vi "Is cancelled.vi"(8 "error in (no error)":errorcluster, 11 "Progress Dialog in":refnum<class "Progress Dialog.lvclass">) -> (0 "error out":errorcluster, 2 "Cancelled?":bool, 3 "Progress Dialog out":refnum<class "Progress Dialog.lvclass">)   [LabVIEW 2011, in "COSYLib.lvlib" / "Progress Dialog.lvclass"]
uses:
  Progress Dialog.lvclass
  Progress Dialog.lvclass/Progress Dialog.ctl
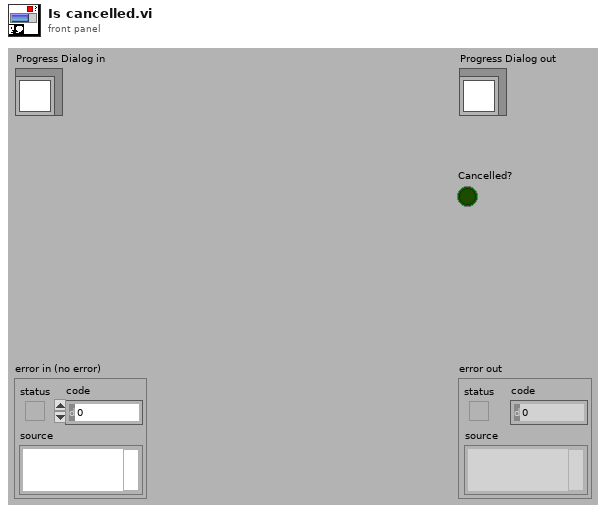
[diagram p1: front panel]
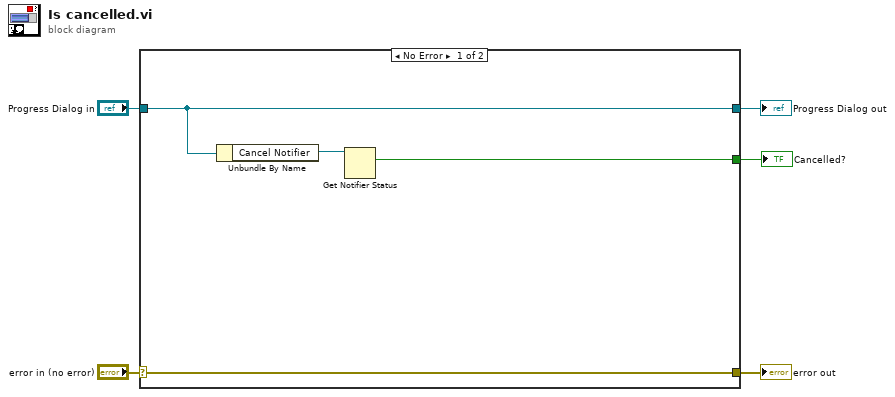
[diagram p0: block diagram]
diagram:
  n1 = case shown="No Error" "error in (no error)" {
    selector: "error in (no error)" -> [w9 w11]
    tunnel: [w9 w11] -> w4
    tunnel: [w8 w10] -> w2
    tunnel: "Progress Dialog in" -> [w8 w10]
    tunnel: [w6 _] -> w1
    frame No Error {
      n2 = Unbundle By Name(w8) -> ("Cancel Notifier"=w7:refnum<notifier>)
      n3 = Get Notifier Status(notifier=w7) -> (current notification=w6:bool)  [unwired: 1 in, 4 out]
    }
    frame Error {
    }
  }
  "error out" <- w4
  "Progress Dialog out" <- w2
  "Cancelled?" <- w1
